vi "GetOutputShapeDim.vi"(7 "DLL path":path, 8 "error in (no error)":errorcluster, 9 "dimIndex":i32, 10 "outputIndex":i32, 11 "session id in":i32) -> (0 "error out":errorcluster, 2 "OutputShapeDim":i64, 3 "session id out":i32)   [LabVIEW 2017, in "ONNX Class Library.lvlib"]
doc: "/**\n * @brief Получить значение конкретной размерности выходного тензора\n * \n * Возвращает размер тензора по указанному измерению.\n * Например, для shape [1, 3, 224, 224]:\n * - dimIndex=0 вернёт 1 (батч)\n * - dimIndex=1 вернёт 3 (каналы)\n * - dimIndex=2 вернёт 224 (высота)\n * - dimIndex=3 вернёт 224 (ширина)\n * \n * @param sessionId [IN] ID сессии\n * @param outputIndex [IN] Индекс входа (0-based)\n * @param dimIndex [IN] Индекс размерности (0-based, от 0 до GetInputShapeDimCount-1)\n * \n * @return int64: Значение размерности (положительное число)\n * @return int64: -1 если сессия не найдена или индексы неверны\n */\nint64_t GetOutputShapeDim(int sessionId, int outputIndex, int dimIndex);"
uses:
  ONNX Class Library.lvlib
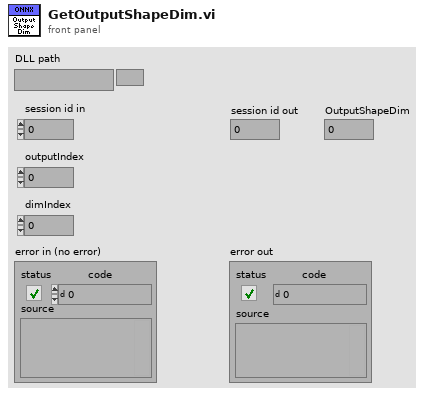
[diagram p1: front panel]
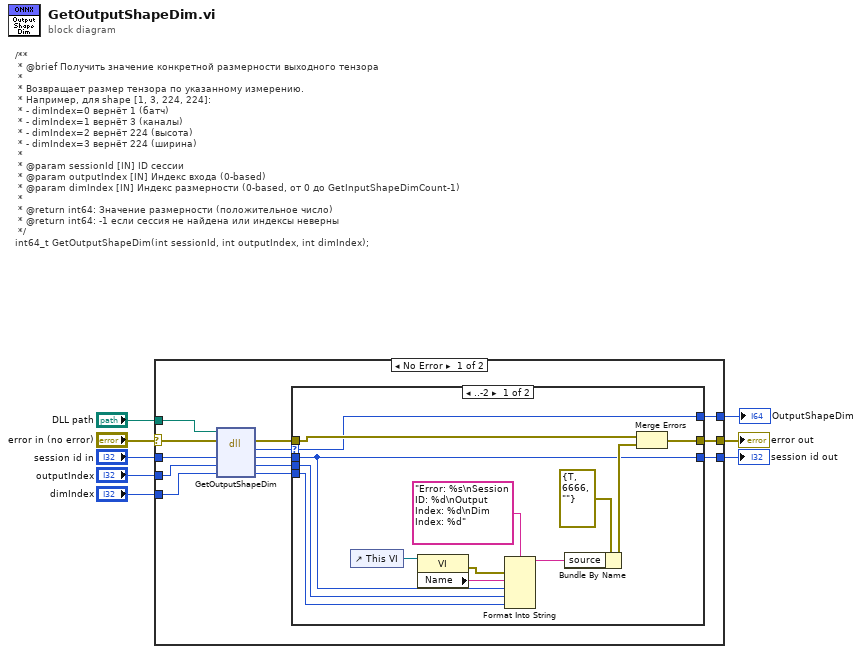
[diagram p0: block diagram]
diagram:
  # "/**\n * @brief Получить значение конкретной размерности выходного тензора\n * \n * Возвращает размер тензора по указанному измерению.\n * Например, для shape [1, 3, 224, 224]:\n * - dimIndex=0 вернёт 1 (батч)\n * - dimIndex=1 вернёт 3 (каналы)\n * - dimIndex=2 вернёт 224 (высота)\n * - dimIndex=3 вернёт 224 (ширина)\n * \n * @param sessionId [IN] ID сессии\n * @param outputIndex [IN] Индекс входа (0-based)\n * @param dimIndex [IN] Индекс размерности (0-based, от 0 до GetInputShapeDimCount-1)\n * \n * @return int64: Значение размерности (положительное число)\n * @return int64: -1 если сессия не найдена или индексы неверны\n */\nint64_t GetOutputShapeDim(int sessionId, int outputIndex, int dimIndex);"
  n1 = case shown="No Error" "error in (no error)" {
    selector: "error in (no error)" -> [w9 w39]
    tunnel: "outputIndex" -> [w21 _]
    tunnel: "session id in" -> [w20 w38]
    tunnel: "dimIndex" -> [w19 _]
    tunnel: [w17 w39] -> w5
    tunnel: [w16 _] -> w4
    tunnel: [w15 w38] -> w3
    tunnel: "DLL path" -> [w10 _]
    frame No Error {
      n2 = dll-call lib="home/ivan/LabVIEWData/ONNX/Test/libonnx_wrapper/unix64/libonnx_wrapper.so" fn="GetOutputShapeDim"(path in=w10, error in=w9, "sessionId"=w20, "outputIndex"=w21, "dimIndex"=w19) -> (error out=w18:errorcluster, "return"=w14:i64, "sessionId"=w13:i32, "outputIndex"=w12:i32, "dimIndex"=w11:i32)  [unwired: 1 in, 1 out]
      n3 = case shown="..-2" w14 {
        selector: w14 -> [w23 w35]
        tunnel: w18 -> [w25 w37]
        tunnel: [w26 w37] -> w17
        tunnel: w13 -> [w27 w36]
        tunnel: [w27 w36] -> w15
        tunnel: w12 -> [w24 _]
        tunnel: [w23 w35] -> w16
        tunnel: w11 -> [w22 _]
        frame ..-2 {
          n4 = control-ref of="This VI"() -> (w31:refnum<vi>)
          n5 = property class="VI"(reference=w31) -> (error out=w28:errorcluster, "Name"=w30:string)  [unwired: 1 in, 1 out]
          n6 = Format Into String(format string="Error: %s\nSession ID: %d\nOutput Index: %d\nDim Index: %d", error in=w28, w30, w27, w24, w22) -> (resulting string=w32:string)  [unwired: 1 in, 1 out]
          n7 = Bundle By Name(cluster=errorcluster {"status"=TRUE, "code"=6666, "source"=""} ("error out"), "source"=w32) -> (w33:errorcluster)
          n8 = Merge Errors(w25, w33) -> (w26:errorcluster)
        }
        frame -1.. {
        }
      }
    }
    frame Error {
    }
  }
  "error out" <- w5
  "session id out" <- w3
  "OutputShapeDim" <- w4
